vi "agentKilled.vi"(1 "Agent ID":string, 2 "killNotifier":refnum<notifier>) -> (0 "Stop":bool)   [LabVIEW 2009, in "MoAgSy.lvlib" / "MoAgSy_Engine.lvclass"]
uses:
  MoAgSy_Engine.lvclass
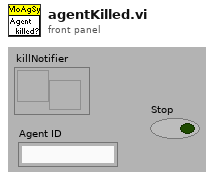
[diagram p1: front panel]
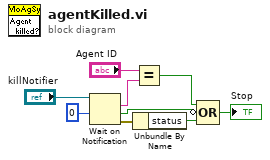
[diagram p0: block diagram]
diagram:
  n1 = Wait on Notification(notifier="killNotifier", timeout in ms (-1)=0) -> (notification=w3:string, timed out?=w5:bool, error out=w7:errorcluster)  [unwired: 1 in, 2 out]
  n2 = Unbundle By Name(w7) -> ("status"=w8:bool)
  n3 = Equal?(x="Agent ID", y=w3) -> (x = y?=w6:bool)
  n4 = Compound Arithmetic op=OR(w6, invert w5, w8) -> (→"Stop":bool)
